vi "Set GObject.vi"(8 "error in (no error)":errorcluster, 10 "GObject.lvclass":refnum<class "GObject.lvclass">, 11 "VI Data in":refnum<class "VI Data.lvclass">) -> (0 "error out":errorcluster, 2 "Replaced?":bool, 3 "VI Data out":refnum<class "VI Data.lvclass">)   [LabVIEW 2013, in "SET Project Data.lvlib" / "VI Data.lvclass"]
uses:
  VI Data.lvclass
  Control Classes/GObject/GObject.lvclass
  VI Data.lvclass/VI Data.ctl
  Control Classes/GObject/Read UID.vi
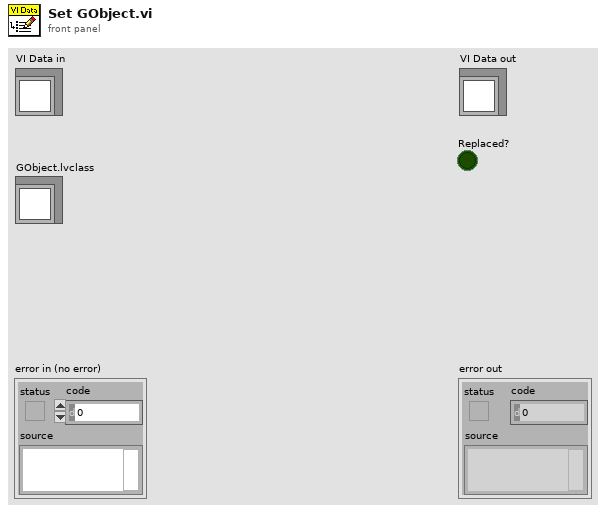
[diagram p1: front panel]
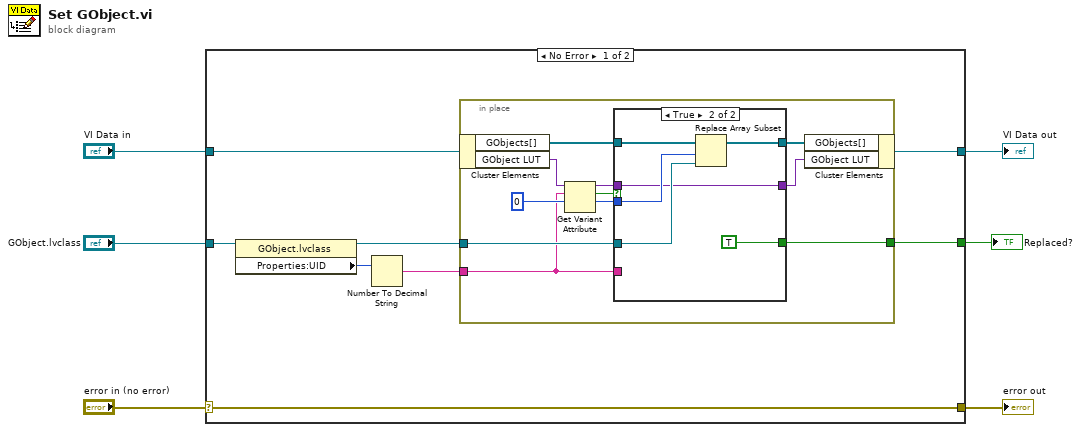
[diagram p0: block diagram]
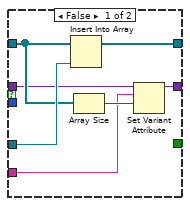
[diagram p2: hidden frame]
diagram:
  n1 = case shown="No Error" "error in (no error)" {
    selector: "error in (no error)" -> [w14 w40]
    tunnel: [w14 w40] -> w5
    tunnel: [w9 w39] -> w3
    tunnel: "VI Data in" -> [w11 w39]
    tunnel: "GObject.lvclass" -> [w13 _]
    tunnel: [w7 _] -> w1
    frame No Error {
      n2 = property class="GObject.lvclass"(reference=w13) -> (reference out=w10:refnum<class "GObject.lvclass">, "Properties:UID"=w12:i32)  [unwired: 1 in, 1 out]
      n3 = Number To Decimal String(number=w12) -> (decimal integer string=w8:string)  [unwired: 1 in]
      n4 = in-place {
        in-place-border: w10 -> [w23]
        in-place-border: w8 -> [w16]
        in-place-border: [w15] -> w7
        n5 = in-place-cluster #1(w11) -> ("GObjects[]"=w25:refnum<class "GObject.lvclass">[], "GObject LUT"=w22:variant)
        n6 = Get Variant Attribute(Variant=w22, name=w16, default value (empty Variant)=0) -> (duplicate Variant=w18:variant, found=w21:bool, value=w19:i32)  [unwired: 1 in, 1 out]
        n7 = case shown="True" w21 {
          tunnel: w25 -> [w30 w38]
          tunnel: [w32 w37] -> w24
          tunnel: w23 -> [w31 w36]
          tunnel: w19 -> [_ w35]
          tunnel: w18 -> [w28 w34]
          tunnel: [w29 w34] -> w17
          tunnel: w16 -> [w26 _]
          tunnel: [_ TRUE] -> w15
          frame False {
            n8 = Insert Into Array(array=w30, new element=w31) -> (w32:refnum<class "GObject.lvclass">[])  [unwired: 1 in]
            n9 = Array Size(array=w30) -> (size(s)=w27:i32)
            n10 = Set Variant Attribute(Variant=w28, name=w26, value=w27) -> (Variant out=w29:variant)  [unwired: 1 in, 2 out]
          }
          frame True {
            n11 = Replace Array Subset(array=w38, new element=w36, index=w35) -> (w37:refnum<class "GObject.lvclass">[])
          }
        }
        n12 = in-place-cluster #1("GObjects[]"=w24, "GObject LUT"=w17) -> (w9:refnum<class "VI Data.lvclass">)
      }
    }
    frame Error {
    }
  }
  "error out" <- w5
  "VI Data out" <- w3
  "Replaced?" <- w1
